vi "Write CombinedConfig.vi"(10 "Combined Config":T1={"ILCAppConfig"={"ILCConfig"={"Input Channels"=enum."Channel 0", "Scan Rate (Hz) "=enum."50", "ADC PGA Gain"=0}, "SerialConfig"={"VISA resource name"="", "Baud Rate"=9600, "Data Bits"=8, "Parity"=enum."None", "Stop Bits"=10, "Flow Control"=0, "Timeout (ms)"=10000, "Serial Protocol"=enum."RS485"}, "Application Timing"={"Loop Period (ms)"=100}}, "Actuator"={"Serial Configurations for Sensors"={"Motor Temperature Sensor"={"VISA resource name"="", "Baud Rate"=9600, "Data Bits"=8, "Parity"=enum."None", "Stop Bits"=10, "Flow Control"=0, "Timeout (ms)"=10000, "Serial Protocol"=enum."RS485"}, "Ambient Temperature Sensor"={"VISA resource name"="", "Baud Rate"=9600, "Data Bits"=8, "Parity"=enum."None", "Stop Bits"=10, "Flow Control"=0, "Timeout (ms)"=10000, "Serial Protocol"=enum."RS485"}, "Distance Gauge"={"VISA resource name"="", "Baud Rate"=9600, "Data Bits"=8, "Parity"=enum."None", "Stop Bits"=10, "Flow Control"=0, "Timeout (ms)"=10000, "Serial Protocol"=enum."RS485"}}, "Stepper Motor"={"Maximum Step Rate"=5000000.0}, "Sensor Data"={"Force Sensor Conversion"=5000.0}, "Controller"={"Per Step Delta Force"=5000.0}, "Exception Stop Conditions"={"Motor Overheat Temperature"=274.15}}} {"Actuator"."Exception Stop Conditions"."Motor Overheat Temperature" min=274.15 max=573.15 format="%.1f"; "Actuator"."Controller"."Per Step Delta Force" min=10.0 max=5000.0; "Actuator"."Sensor Data"."Force Sensor Conversion" min=0.01 max=5000.0 format="%.2f"; "Actuator"."Stepper Motor"."Maximum Step Rate" min=10000.0 max=5000000.0; "Actuator"."Serial Configurations for Sensors"."Distance Gauge"."Stop Bits" items=["1.0"=10, "1.5"=15, "2.0"=20]; "Actuator"."Serial Configurations for Sensors"."Distance Gauge"."Flow Control" items=["None", "XON/XOFF", "RTS/CTS", "XON/XOFF & RTS/CTS", "DTR/DSR", "XON/XOFF & DTR/DSR"]; "Actuator"."Serial Configurations for Sensors"."Distance Gauge"."Data Bits" min=5 max=8 step=1; "Actuator"."Serial Configurations for Sensors"."Ambient Temperature Sensor"."Stop Bits" items=["1.0"=10, "1.5"=15, "2.0"=20]; "Actuator"."Serial Configurations for Sensors"."Ambient Temperature Sensor"."Flow Control" items=["None", "XON/XOFF", "RTS/CTS", "XON/XOFF & RTS/CTS", "DTR/DSR", "XON/XOFF & DTR/DSR"]; "Actuator"."Serial Configurations for Sensors"."Ambient Temperature Sensor"."Data Bits" min=5 max=8 step=1; "Actuator"."Serial Configurations for Sensors"."Motor Temperature Sensor"."Stop Bits" items=["1.0"=10, "1.5"=15, "2.0"=20]; "Actuator"."Serial Configurations for Sensors"."Motor Temperature Sensor"."Flow Control" items=["None", "XON/XOFF", "RTS/CTS", "XON/XOFF & RTS/CTS", "DTR/DSR", "XON/XOFF & DTR/DSR"]; "Actuator"."Serial Configurations for Sensors"."Motor Temperature Sensor"."Data Bits" min=5 max=8 step=1; "ILCAppConfig"."Application Timing"."Loop Period (ms)" min=1 max=5000; "ILCAppConfig"."SerialConfig"."Stop Bits" items=["1.0"=10, "1.5"=15, "2.0"=20]; "ILCAppConfig"."SerialConfig"."Flow Control" items=["None", "XON/XOFF", "RTS/CTS", "XON/XOFF & RTS/CTS", "DTR/DSR", "XON/XOFF & DTR/DSR"]; "ILCAppConfig"."SerialConfig"."Data Bits" min=5 max=8 step=1; "ILCAppConfig"."ILCConfig"."ADC PGA Gain" max=7}, 11 "Start in":refnum<class "Start.lvclass">) -> (3 "Start out":refnum<class "Start.lvclass">)   [LabVIEW 2013, in "Start.lvclass"]
uses:
  Start.lvclass
  Configuration/Combined Config.ctl
  Configuration/ILCAppConfig.ctl
  <userlib>/Common/ILC/Configuration/ILCConfig.ctl
  <userlib>/Common/ILC/Configuration/InputChannels.ctl
  <userlib>/Common/ILC/Configuration/ScanRate_Hz_MultichannelOptions.ctl
  <userlib>/Common/SerialProtocols/Configuration/SerialConfig.ctl
  <userlib>/Common/SerialProtocols/Configuration/SerialProtocol.ctl
  <userlib>/Common/Component/Application/Configuration/ApplicationTiming.ctl
  Configuration/Actuator.ctl
  Configuration/Serial Configuration For Sensors.ctl
  Configuration/Stepper Motor.ctl
  Configuration/SensorData.ctl
  Configuration/Controller.ctl
  Configuration/ExceptionStopConditions.ctl
  Start.lvclass/Start.ctl
  <userlib>/Common/ILC/Configuration/ILCConfiguration.lvlib
  <userlib>/Common/SerialProtocols/SerialProtocols.lvlib
  <userlib>/Common/Component/Application/Application.lvlib
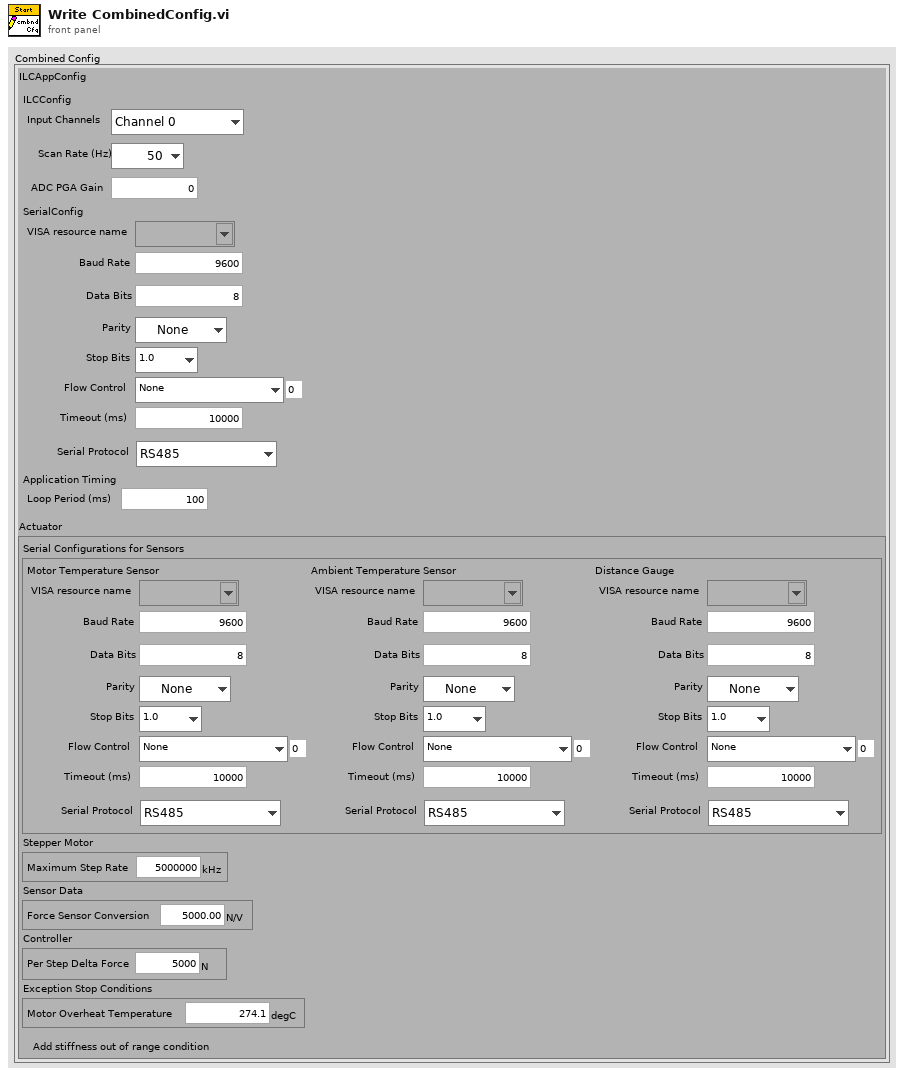
[diagram p1: front panel]
types:
  T1 = typedef "Combined Config.ctl" = cluster{"ILCAppConfig":T2, "Actuator":T9}
  T2 = typedef "ILCAppConfig.ctl" = cluster{"ILCConfig":T3, "SerialConfig":T6, "Application Timing":T8}
  T3 = typedef "ILCCommon.lvlib/ILCConfiguration.lvlib/ILCConfig.ctl" = cluster{"Input Channels":T4, "Scan Rate (Hz) ":T5, "ADC PGA Gain":u8}
  T4 = typedef "ILCCommon.lvlib/ILCConfiguration.lvlib/InputChannels.ctl" = enum16{"Channel 0", "3 Channels", "5 Channels"}
  T5 = typedef "ILCCommon.lvlib/ILCConfiguration.lvlib/ScanRate_Hz_MultichannelOptions.ctl" = enum16{"50", "60", "100", "120", "200", "240", "300", "400", "480", "600", "1200", "2400", "4800"}
  T6 = typedef "SerialProtocols.lvlib/SerialConfig.ctl" = cluster{"VISA resource name":refnum<visa-resource-name>, "Baud Rate":u32, "Data Bits":u16, "Parity":enum16{"None", "Odd", "Even", "Mark", "Space"}, "Stop Bits":u16, "Flow Control":u16, "Timeout (ms)":u32, "Serial Protocol":T7}
  T7 = typedef "SerialProtocols.lvlib/SerialProtocol.ctl" = enum16{"RS232", "RS485", "SerialSimulator"}
  T8 = typedef "Application.lvlib/ApplicationTiming.ctl" = cluster{"Loop Period (ms)":u16}
  T9 = typedef "Actuator.ctl" = cluster{"Serial Configurations for Sensors":T10, "Stepper Motor":T11, "Sensor Data":T12, "Controller":T13, "Exception Stop Conditions":T14}
  T10 = typedef "Serial Configuration For Sensors.ctl" = cluster{"Motor Temperature Sensor":T6, "Ambient Temperature Sensor":T6, "Distance Gauge":T6}
  T11 = typedef "Stepper Motor.ctl" = cluster{"Maximum Step Rate":dbl[unit]}
  T12 = typedef "SensorData.ctl" = cluster{"Force Sensor Conversion":dbl[unit]}
  T13 = typedef "Controller.ctl" = cluster{"Per Step Delta Force":dbl[unit]}
  T14 = typedef "ExceptionStopConditions.ctl" = cluster{"Motor Overheat Temperature":dbl[unit]}
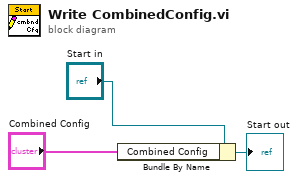
[diagram p0: block diagram]
diagram:
  n1 = Bundle By Name(cluster="Start in", "Combined Config"="Combined Config") -> (→"Start out":refnum<class "Start.lvclass">)
